vi "GPS Map Graph.vi"(5 "Path to configuration":path=path "E:/Dropbox/Condivise/Condivisa con Fausto Petruzzelli/Test/GPS/Test_gps_3/mappa1.txt", 7 "Path to Image":path=path "E:/Dropbox/Condivise/Condivisa con Fausto Petruzzelli/Test/GPS/Test_gps_3/mappa1.png", 8 "Error In":errorcluster, 9 "Function":T1, 10 "Coordinate":cluster{"Latitudine":dbl, "Longitudine":dbl}, 11 "Map":refnum<vi>) -> (0 "Error Out":errorcluster, 3 "Map":cluster{"X":dbl, "Y":dbl}[](graph))   [LabVIEW 2013]
uses:
  Gps Map Graph enum.ctl
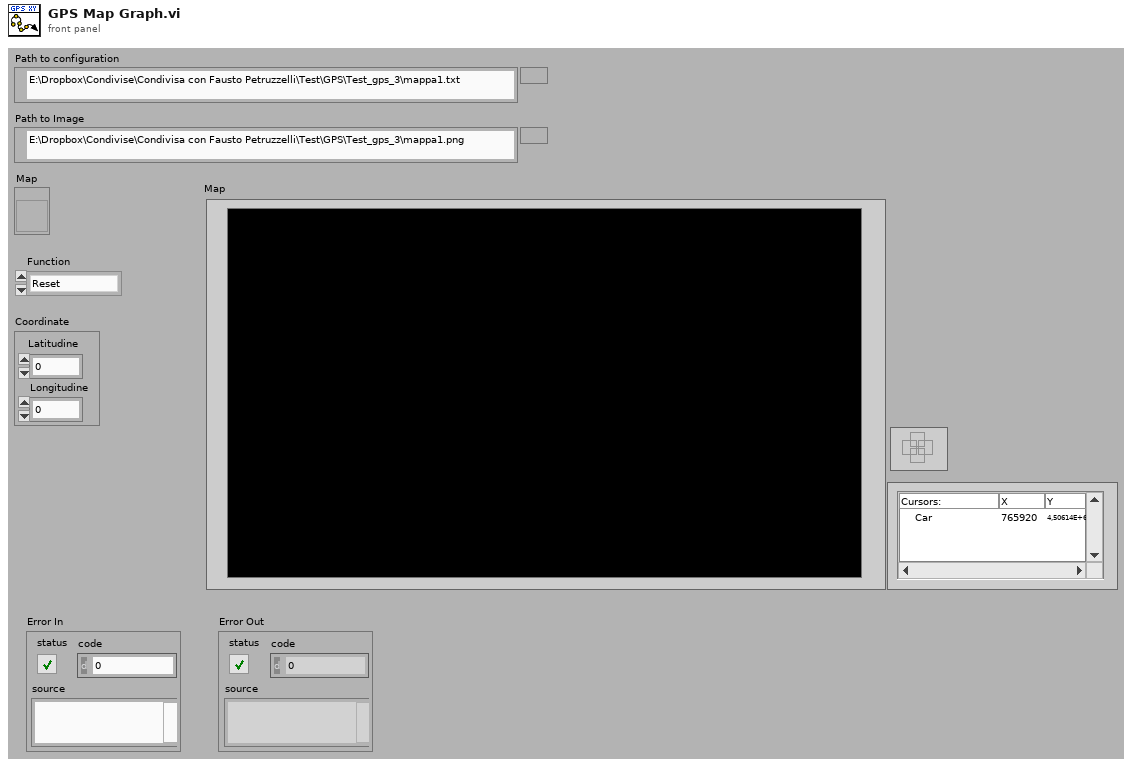
[diagram p1: front panel]
types:
  T1 = typedef "Gps Map Graph enum.ctl" = enum16{"Reset", "SetValue"}
  T2 = cluster{"Top":dbl, "Bottom":dbl, "Right":dbl, "Left":dbl}
  T3 = enum16{"open", "replace", "create", "open or create", "replace or create", "replace or create with confirmation"}
  T4 = typedef "imagedata.ctl" = cluster{"image type":i32, "image depth":i32, "image":u8[], "mask":u8[], "colors":u32[], "Rectangle":cluster{"left":i16, "top":i16, "right":i16, "bottom":i16}}
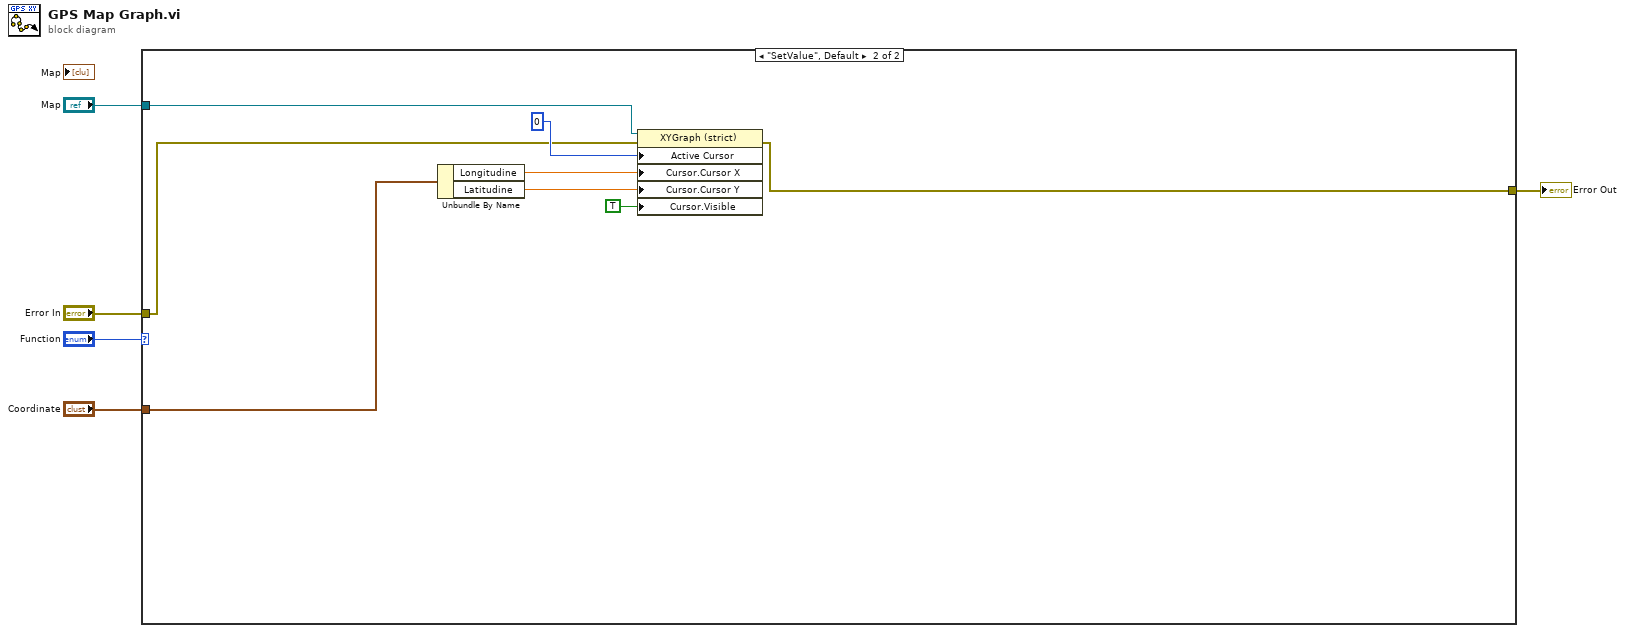
[diagram p0: block diagram]
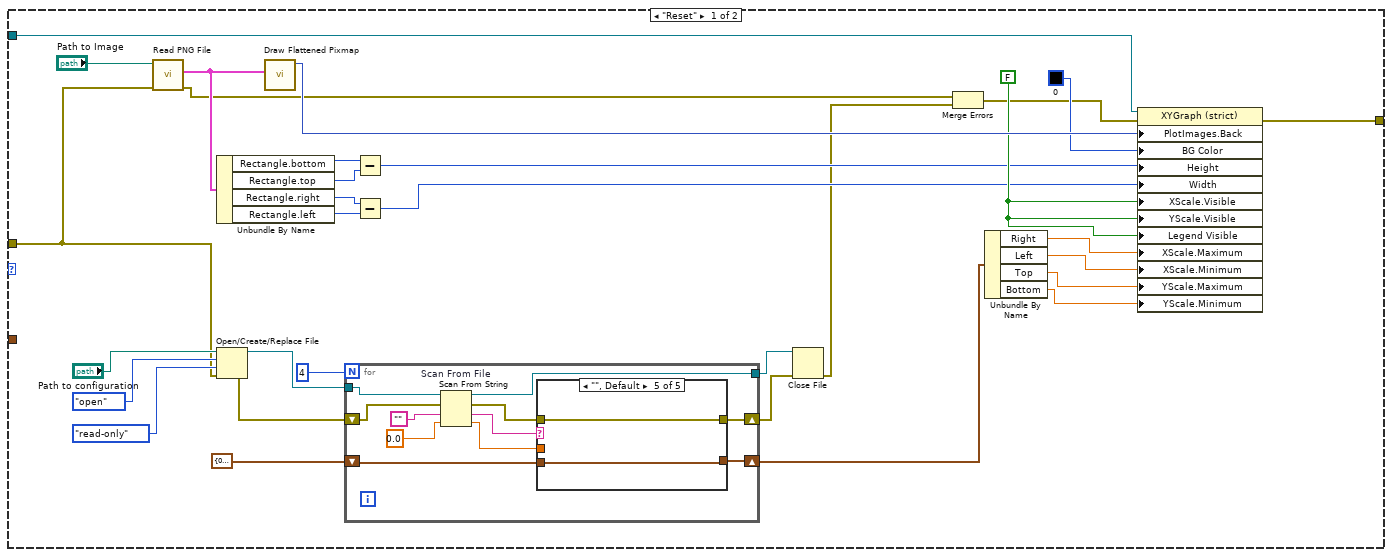
[diagram p2: hidden frame]
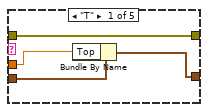
[diagram p3: hidden frame]
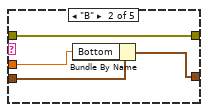
[diagram p4: hidden frame]
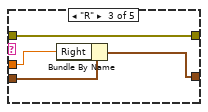
[diagram p5: hidden frame]
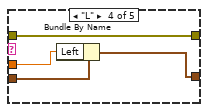
[diagram p6: hidden frame]
diagram:
  n1 = case shown="\"SetValue\", Default" "Function" {
    tunnel: [w8 w70] -> w5
    tunnel: "Error In" -> [w7 w71]
    tunnel: "Map" -> [w6 w72]
    tunnel: "Coordinate" -> [_ w69]
    frame "Reset" {
      w33 = FALSE ("X Scale.Visible")
      n2 = call <vilib>:"Read PNG File.vi"("error in (no error)"=w7, "path to PNG file"="Path to Image") -> ("error out"=w9:errorcluster, "image data"=w32:T4)  [unwired: 7 in, 1 out]
      n3 = Unbundle By Name(w32) -> ("Rectangle.bottom"=w31:i16, "Rectangle.top"=w30:i16, "Rectangle.right"=w29:i16, "Rectangle.left"=w28:i16)
      n4 = Open/Create/Replace File(file path (use dialog)="Path to configuration", error in=w7, operation (0:open)=T3."open", access (0:read/write)=enum16{"read/write", "read-only", "write-only"}."read-only") -> (refnum out=w22:refnum<file>, error out=w21:errorcluster)  [unwired: 2 in, 1 out]
      n5 = call <vilib>:"Draw Flattened Pixmap.vi"("image data"=w32) -> ("new picture"=w36:picture)  [unwired: 8 in]
      n6 = for {
        N: 4 -> [_]
        tunnel: w22 -> [w47]
        shift-right: [w40] -> w16
        shift-left: T2 {"Top"=0.0, "Bottom"=0.0, "Right"=0.0, "Left"=0.0} -> [w41]
        shift-right: [w39] -> w18
        shift-left: w21 -> [w46]
        tunnel: [w38] -> w17
        n7 = Scan From String "Scan From File"(w47, w46, default 1="", default 2=0.0) -> (w38:refnum<file>, w42:errorcluster, output 1=w44:string, output 2=w43:dbl)  [unwired: 1 in]
        n8 = case shown="\"\", Default" w44 {
          tunnel: w43 -> [w50 w53 w57 w61 _]
          tunnel: w42 -> [w48 w55 w59 w63 w65]
          tunnel: w41 -> [w51 w54 w58 w62 w64]
          tunnel: [w49 w52 w56 w60 w64] -> w40
          tunnel: [w48 w55 w59 w63 w65] -> w39
          frame "T" {
            n9 = Bundle By Name(cluster=w51, "Top"=w50) -> (w49:T2)
          }
          frame "B" {
            n10 = Bundle By Name(cluster=w54, "Bottom"=w53) -> (w52:T2)
          }
          frame "R" {
            n11 = Bundle By Name(cluster=w58, "Right"=w57) -> (w56:T2)
          }
          frame "L" {
            n12 = Bundle By Name(cluster=w62, "Left"=w61) -> (w60:T2)
          }
          frame "", Default {
          }
        }
      }
      n13 = Subtract(x=w31, y=w30) -> (x-y=w27:i16)
      n14 = Subtract(x=w29, y=w28) -> (x-y=w26:i16)
      n15 = Close File(refnum=w17, error in=w18) -> (error out=w10:errorcluster)  [unwired: 1 out]
      n16 = Merge Errors(w9, w10) -> (w11:errorcluster)
      n17 = Unbundle By Name(w16) -> ("Right"=w12:dbl, "Left"=w13:dbl, "Top"=w14:dbl, "Bottom"=w15:dbl)
      n18 = property on="Property Node" class="XYGraph (strict)"(reference=w6, error in=w11, "PlotImages.Back"=w36, "BG Color"=u32 0, "Height"=w27, "Width"=w26, "XScale.Visible"=w33, "YScale.Visible"=w33, "Legend Visible"=w33, "XScale.Maximum"=w12, "XScale.Minimum"=w13, "YScale.Maximum"=w14, "YScale.Minimum"=w15) -> (error out=w8:errorcluster)  [unwired: 1 out]
    }
    frame "SetValue", Default {
      n19 = Unbundle By Name(w69) -> ("Longitudine"=w68:dbl, "Latitudine"=w67:dbl)
      n20 = property class="XYGraph (strict)"(reference=w72, error in=w71, "Active Cursor"=u32 0, "Cursor.Cursor X"=w68, "Cursor.Cursor Y"=w67, "Cursor.Visible"=TRUE) -> (error out=w70:errorcluster)  [unwired: 1 out]
    }
  }
  "Error Out" <- w5
